vi "Initialize FPGA Starter Kit Host.vi"(7 "run FPGA (T)":bool=TRUE, 8 "error in (no error)":errorcluster, 10 "IP address (\"\")":string, 11 "FPGA starter kit host in":refnum<class "NI_Robotics_Starter Kit Host_FPGA_2.0.lvclass">) -> (0 "error out":errorcluster, 3 "FPGA starter kit host out":refnum<class "NI_Robotics_Starter Kit Host_FPGA_2.0.lvclass">)   [LabVIEW 2017, in "NI_Robotics_Starter Kit Host_FPGA_2.0.lvclass"]
uses:
  <vilib>/robotics/Starter Kit/2.0/FPGA Host Interface/NI_Robotics_Starter Kit Host_FPGA_2.0.lvclass
  c:/Program Files (x86)/National Instruments/LabVIEW 2017/vi.lib/robotics/Starter Kit/Host Interface/NI_Robotics_Starter Kit Host.lvclass
  <vilib>/robotics/Starter Kit/2.0/FPGA Host Interface/NI_Robotics_Starter Kit Host_FPGA_2.0.lvclass/NI_Robotics_Starter Kit Host_FPGA_2.0.ctl
  <vilib>/robotics/Starter Kit/Host Interface/NI_Robotics_Starter Kit Host.lvclass/NI_Robotics_Starter Kit Host.ctl
  <vilib>/robotics/Starter Kit/FPGA Direct IO/NI_Robotics_Starter Kit Direct IO_FPGA.lvclass/NI_Robotics_Starter Kit Direct IO_FPGA.ctl
  <vilib>/robotics/Starter Kit/Base Device/NI_Robotics_Starter Kit Base Device.lvclass/NI_Robotics_Starter Kit Base Device.ctl
  <vilib>/robotics/Starter Kit/Host Interface/Set DC Motors.vi
  <vilib>/robotics/Starter Kit/Host Interface/Set PING))) Sensor.vi
  <vilib>/robotics/Starter Kit/Host Interface/Set Sensor Servo.vi
  <vilib>/robotics/Starter Kit/FPGA Direct IO/Create FPGA Direct IO.vi
  <vilib>/robotics/Starter Kit/Host Interface/Set Direct IO.vi
  <vilib>/robotics/Starter Kit/Host Interface/Mark Initialized.vi
  <vilib>/robotics/Starter Kit/Base Device/Mark Initialized.vi
  <vilib>/robotics/Starter Kit/Servo Motor 2.0/NI_Robotics_Starter Kit Servo Motor_2.0.lvclass
  c:/Program Files (x86)/National Instruments/LabVIEW 2017/vi.lib/robotics/Starter Kit/Servo Motor/NI_Robotics_Starter Kit Servo Motor.lvclass
  <vilib>/robotics/Starter Kit/FPGA Direct IO/NI_Robotics_Starter Kit Direct IO_FPGA.lvclass
  c:/Program Files (x86)/National Instruments/LabVIEW 2017/vi.lib/robotics/Starter Kit/Base Device/NI_Robotics_Starter Kit Base Device.lvclass
  c:/Program Files (x86)/National Instruments/LabVIEW 2017/vi.lib/robotics/Starter Kit/Direct IO/NI_Robotics_Starter Kit Direct IO.lvclass
  <vilib>/robotics/Starter Kit/Servo Motor 2.0/Create 2.0 Servo Motor.vi
  <instrlib>/Hitec HS400 Series/HAIOL/FPGA/Public/Initialize (FPGA).vi
  <instrlib>/Parallax PING)))/HAIOL/FPGA/Public/Initialize (FPGA).vi
  <instrlib>/DC Motor Controller/HAIOL/FPGA/Public/Initialize (FPGA).vi
  <vilib>/FPGAPlugInAG/Dynamic/niLvFpga_Run_Dynamic.vi
  <vilib>/robotics/Starter Kit/2.0/FPGA Host Interface/FPGA Refnum.ctl
  <vilib>/rvi/interface/nirviMethod/nirviMethod.xnode
  <vilib>/robotics/Starter Kit/FPGA Host Interface/NI_Robotics_Starter Kit Host_FPGA.lvclass
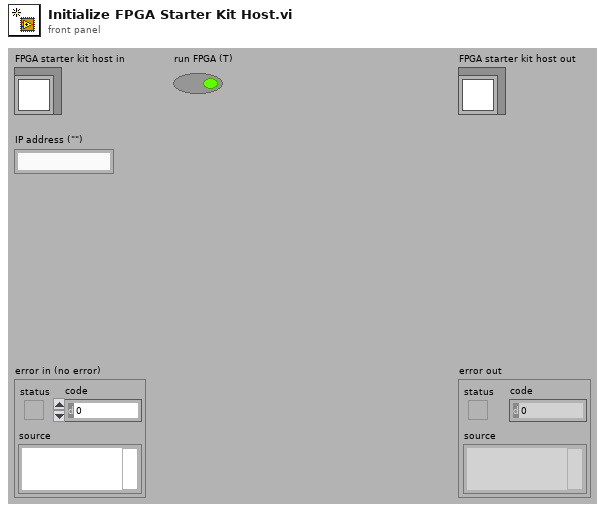
[diagram p1: front panel]
types:
  T1 = typedef "NI_Robotics_Starter Kit Host_FPGA_2.0.lvclass/FPGA Refnum.ctl" = refnum<k20>
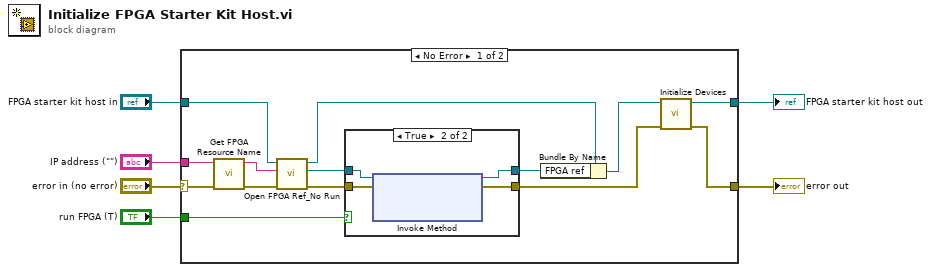
[diagram p0: block diagram]
diagram:
  n1 = case shown="No Error" "error in (no error)" {
    selector: "error in (no error)" -> [w20 w28]
    tunnel: [w7 w28] -> w2
    tunnel: "IP address (\"\")" -> [w19 _]
    tunnel: [w8 w27] -> w3
    tunnel: "FPGA starter kit host in" -> [w13 w27]
    tunnel: "run FPGA (T)" -> [w18 _]
    frame No Error {
      n2 = call <vilib>:"Get FPGA Resource Name.vi"("error in (no error)"=w20, "IP address"=w19) -> ("error out"=w15:errorcluster, "resource name"=w14:string)  [unwired: 8 in]
      n3 = call-dynamic "Open FPGA Ref_No Run.vi"("error in (no error)"=w15, "resource name"=w14, "starter kit host 2.0 in"=w13) -> ("error out"=w17:errorcluster, "FPGA Interface"=w16:T1, "starter kit host 2.0 out"=w12:refnum<class "NI_Robotics_Starter Kit Host_FPGA_2.0.lvclass">)  [unwired: 6 in]
      n4 = case shown="True" w18 {
        tunnel: [w21 w26] -> w11
        tunnel: w16 -> [w21 w25]
        tunnel: w17 -> [w22 w24]
        tunnel: [w22 w23] -> w9
        frame False {
        }
        frame True {
          n5 = xnode "Invoke Method"("FPGA VI Reference In"=w25, "error in"=w24) -> ("FPGA VI Reference Out"=w26:T1, "error out"=w23:errorcluster)  [unwired: 1 in]
        }
      }
      n6 = Bundle By Name(cluster=w12, "FPGA ref"=w11) -> (w10:refnum<class "NI_Robotics_Starter Kit Host_FPGA_2.0.lvclass">)
      n7 = call <vilib>:"Initialize Devices.vi"("error in (no error)"=w9, "Starter Kit host FPGA 2.0 in"=w10) -> ("error out"=w7:errorcluster, "Starter Kit host FPGA 2.0 out"=w8:refnum<class "NI_Robotics_Starter Kit Host_FPGA_2.0.lvclass">)  [unwired: 8 in]
    }
    frame Error {
    }
  }
  "error out" <- w2
  "FPGA starter kit host out" <- w3
